vi "Avantes - take measurement.vi"(8 "error in (no error)":errorcluster, 10 "UI":refnum<queue>, 11 "Hardware Resources in":T1) -> (0 "error out":errorcluster, 2 "Spectral distribution out":cluster{dbl, dbl}[](graph), 3 "Hardware Resources out":T1)   [LabVIEW 2014, in "AvaSpec.lvlib" / "AvaSpec Acquisition.lvlib"]
doc: "Communicates the the spectrometer to perform measurements. The signal is sent to take a measurement with the corresponding measurement settings. The buffer is then polled for completed measurement data. Raw data is interpolated for integer frequencies, dark corrected, and analyzed for sensor saturation. If the full scale of the sensor isn't utilized optimally a more optimal integration time is itterated over. Once a measurement is taken that optimally uses the sensor range, the spectral distribution is outputted."
uses:
  AvaSpec Acquisition.lvlib
  Hardware Configuration.ctl
  Libraries/AS-5216-DLL/AVS settings.ctl
  Sphere Indicator.ctl
  Settings/Measurement Type.ctl
  support/Message Queue/Message Cluster.ctl
  support/Message Queue/Enqueue Message (Single).vi
  Libraries/AS-5216-DLL/Avantes Spectrometer Functions.lvlib
  support/Message Queue/AvaSpec Message Queue.lvlib
  Dark/Dark.lvlib
  AvaSpec.lvlib
panel:
  out "Raw Spectral distribution":cluster{dbl, dbl}[](graph)
  in  "force stop":bool
  out "i":i32
  # "Inputs"
  # "Out"
  # "Working"
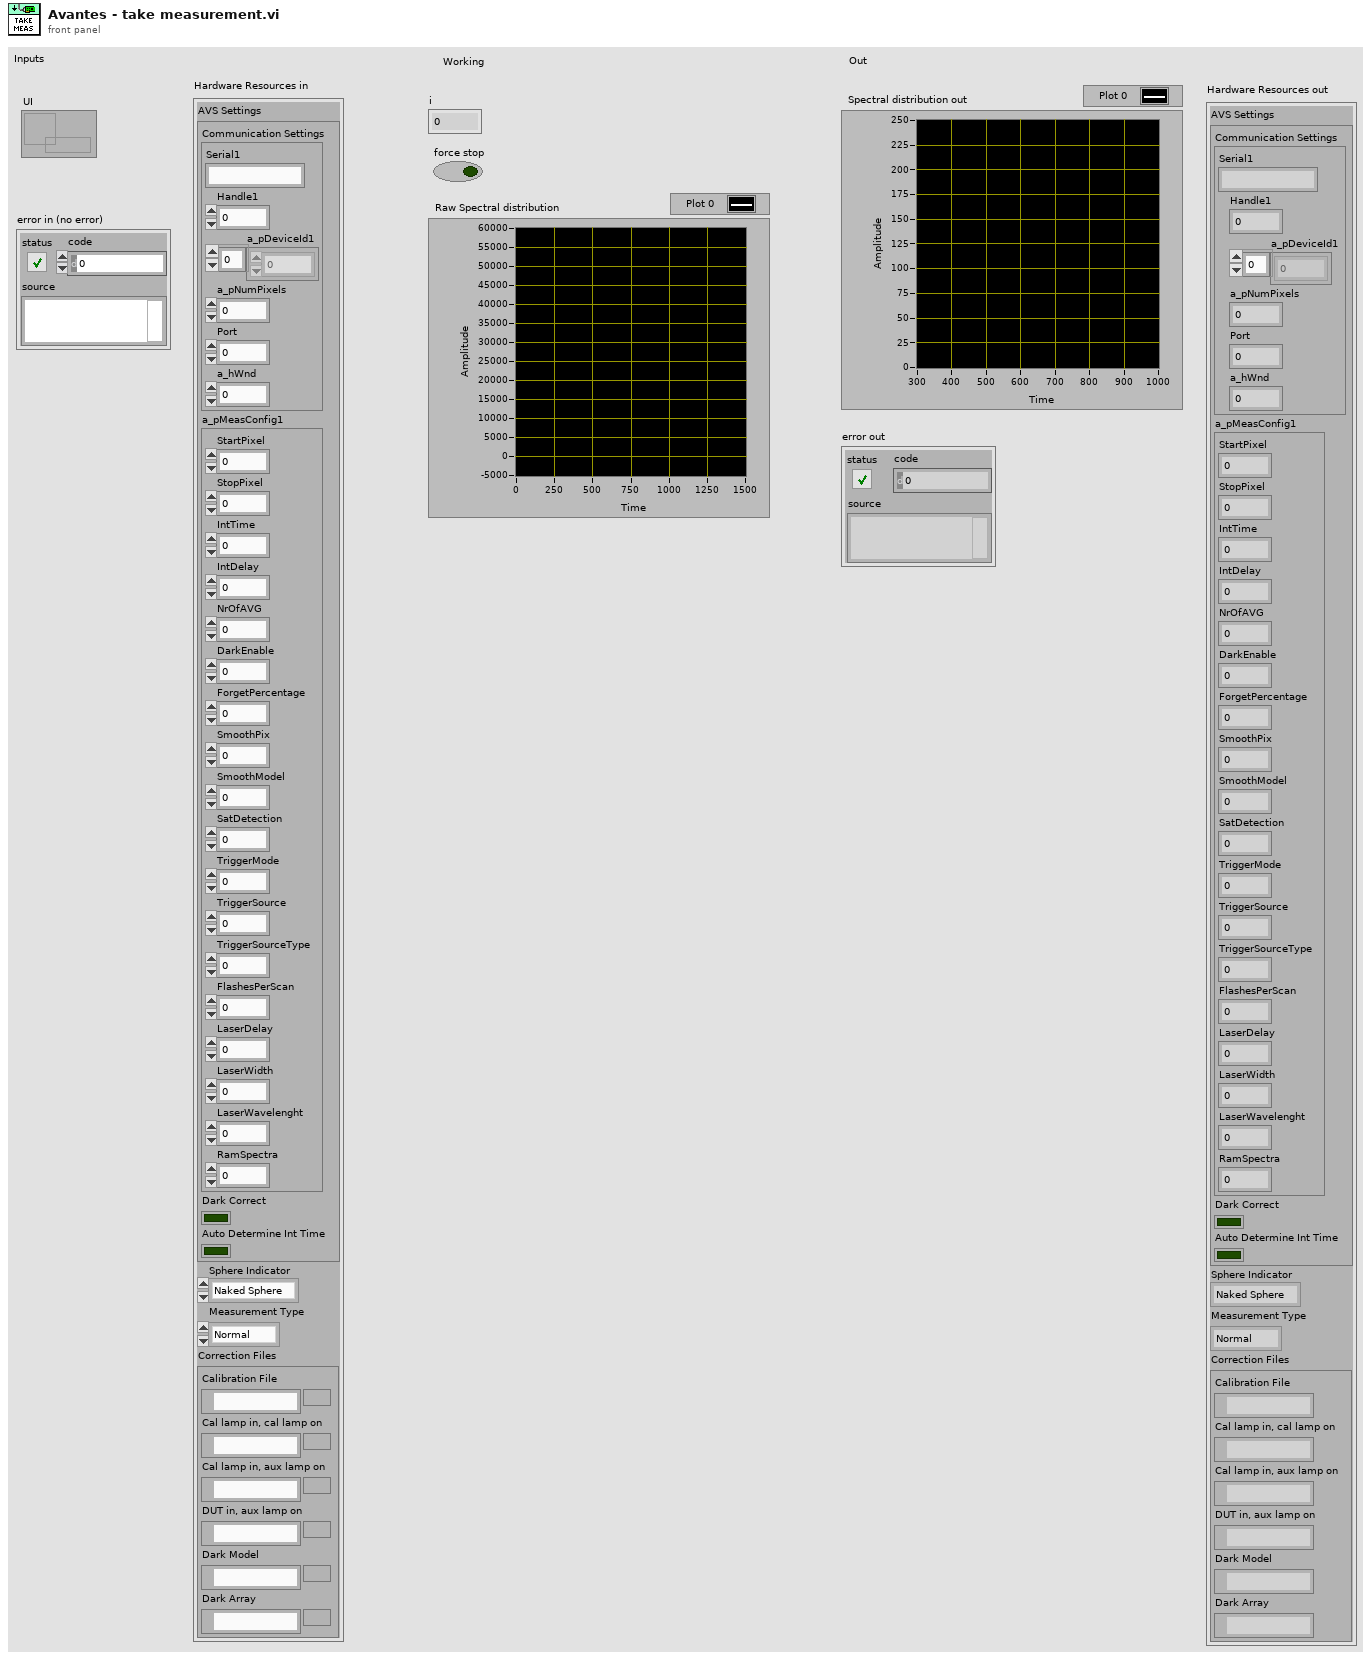
[diagram p1: front panel]
types:
  T1 = typedef "AvaSpec.lvlib/AvaSpec Acquisition.lvlib/Hardware Configuration.ctl" = cluster{"AVS Settings":T2, "Sphere Indicator":T3, "Measurement Type":T4, "Correction Files":cluster{"Calibration File":path, "Cal lamp in, cal lamp on":path, "Cal lamp in, aux lamp on":path, "DUT in, aux lamp on":path, "Dark Model":path, "Dark Array":path}}
  T2 = typedef "AvaSpec.lvlib/AVS settings.ctl" = cluster{"Communication Settings":cluster{"Serial1":string, "Handle1":i32, "a_pDeviceId1":u8[], "a_pNumPixels":u16, "Port":i32, "a_hWnd":i32}, "a_pMeasConfig1":cluster{"StartPixel":u16, "StopPixel":u16, "IntTime":sgl, "IntDelay":u32, "NrOfAVG":u32, "DarkEnable":u8, "ForgetPercentage":u8, "SmoothPix":u16, "SmoothModel":u8, "SatDetection":u8, "TriggerMode":u8, "TriggerSource":u8, "TriggerSourceType":u8, "FlashesPerScan":u16, "LaserDelay":u32, "LaserWidth":u32, "LaserWavelenght":sgl, "RamSpectra":u16}, "Dark Correct":bool, "Auto Determine Int Time":bool}
  T3 = typedef "AvaSpec.lvlib/Sphere Indicator.ctl" = enum16{"Naked Sphere", "Insulated Sphere"}
  T4 = typedef "AvaSpec.lvlib/AvaSpec Acquisition.lvlib/Measurement Type.ctl" = enum16{"Normal", "Calibration", "Dark"}
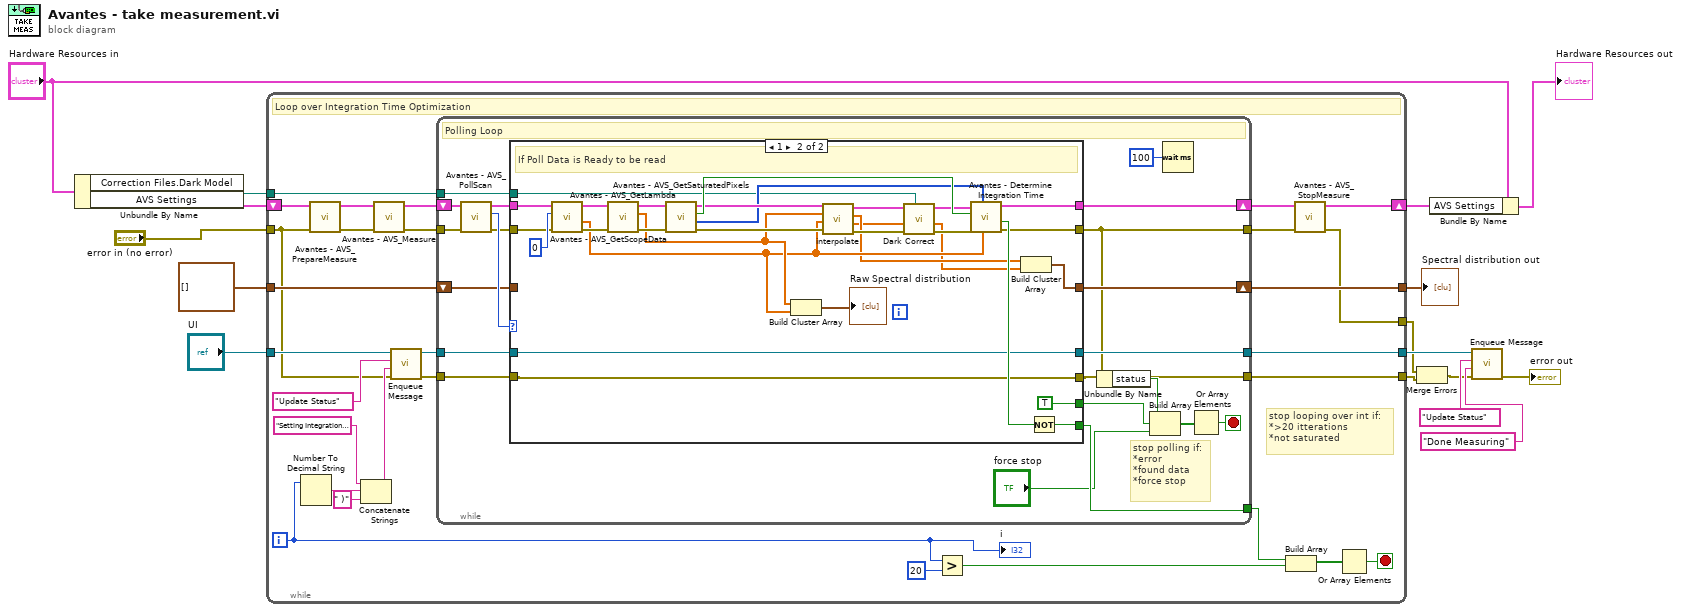
[diagram p0: block diagram]
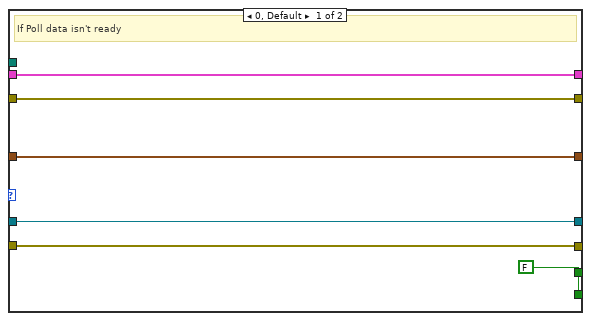
[diagram p2: hidden frame]
diagram:
  n1 = Unbundle By Name("Hardware Resources in") -> ("Correction Files.Dark Model"=w2:path, "AVS Settings"=w8:T2)
  n2 = while {
    tunnel: [w39] -> w4
    tunnel: [w45] -> w16
    tunnel: cluster{dbl, dbl}[] [] -> [w44]
    tunnel: "error in (no error)" -> [w19]
    shift-right: [w40] -> w6
    shift-left: w8 -> [w38]
    tunnel: "UI" -> [w33]
    tunnel: [w25] -> w12
    tunnel: w2 -> [w20]
    tunnel: [w17] -> w3
    i -> [w31]
    stop <- w21 stop-if-true
    # "stop looping over int if:\n*>20 itterations\n*not saturated"
    # "Loop over Integration Time Optimization"
    n3 = Number To Decimal String(number=w31) -> (decimal integer string=w29:string)  [unwired: 1 in]
    n4 = call "Avantes - AVS_PrepareMeasure.vi"("error in (no error)"=w19, "AVS Settings In"=w38) -> ("error out"=w36:errorcluster, "AVS Settings Out"=w37:T2)  [unwired: 8 in]
    n5 = Concatenate Strings("Setting Integration time ( " ("Message"), w29, " )" ("string")) -> (w27:string)
    n6 = call "Avantes - AVS_Measure.vi"("error in (no error)"=w36, "AVS Settings In"=w37) -> ("error out"=w35:errorcluster, "AVS Settings Out"=w34:T2)  [unwired: 8 in]
    n7 = call-poly "Enqueue Message.vi"("error in (no error)"=w19, "Message Data"=w27, "Message"="Update Status", "Message Queue"=w33) -> ("error out"=w18:errorcluster, "dup Message Queue"=w26:refnum<queue>)  [unwired: 6 in]
    n8 = while {
      tunnel: [w51] -> w41
      shift-right: [w63] -> w45
      shift-left: w44 -> [w61]
      shift-right: [w60] -> w43
      shift-left: w34 -> [w57]
      tunnel: [w59] -> w24
      tunnel: w35 -> [w58]
      tunnel: w26 -> [w56]
      tunnel: [w55] -> w25
      tunnel: w20 -> [w48]
      tunnel: w18 -> [w47]
      tunnel: [w46] -> w17
      stop <- w49 stop-if-true
      # "stop polling if:\n*error\n*found data\n*force stop"
      # "Polling Loop"
      n9 = call "Avantes - AVS_PollScan.vi"("error in (no error)"=w58, "AVS Settings In"=w57) -> ("error out"=w64:errorcluster, "Output Ready"=w66:i32, "AVS Settings Out"=w65:T2)  [unwired: 7 in]
      n10 = case shown="1" w66 {
        tunnel: w65 -> [w71 w81]
        tunnel: w64 -> [w72 w101]
        tunnel: [w72 w84] -> w51
        tunnel: [w70 w83] -> w63
        tunnel: [w69 TRUE] -> w52
        tunnel: [w71 w100] -> w60
        tunnel: w61 -> [w70 _]
        tunnel: [w69 w96] -> w59
        tunnel: w56 -> [w68 w95]
        tunnel: [w68 w95] -> w55
        tunnel: w48 -> [_ w87]
        tunnel: [w67 w82] -> w46
        tunnel: w47 -> [w67 w82]
        frame 0, Default {
          w69 = FALSE
          # "If Poll data isn't ready"
        }
        frame 1 {
          # "If Poll Data is Ready to be read"
          n11 = call "Avantes - AVS_GetScopeData.vi"("error in (no error)"=w101, "a_pTimeLabel"=u32 0, "AVS Settings In"=w81) -> ("error out"=w92:errorcluster, "a_pSpectrum"=w77:dbl[], "AVS Settings Out"=w80:T2)  [unwired: 5 in, 1 out]
          n12 = call "Avantes - AVS_GetLambda.vi"("error in (no error)"=w92, "AVS Settings In"=w80) -> ("error out"=w91:errorcluster, "a_pWaveLength"=w78:dbl[], "AVS Settings Out"=w79:T2)  [unwired: 7 in]
          n13 = call "Avantes - AVS_GetSaturatedPixels.vi"("error in (no error)"=w91, "AVS Settings In"=w79) -> ("error out"=w94:errorcluster, "a_pSaturated"=w89:u8[], "Saturated?"=w99:bool, "AVS Settings Out"=w90:T2)  [unwired: 6 in]
          n14 = Build Cluster Array(w78, w77) -> (→"Raw Spectral distribution":cluster{dbl, dbl}[])
          n15 = call "interpolate.vi"("error in (no error)"=w94, "a_pSpectrum"=w77, "a_pWaveLength"=w78, "AVS Settings In"=w90) -> ("error out"=w93:errorcluster, "Counts Out"=w74:dbl[], "Wavelengths Out"=w76:dbl[], "AVS Settings out"=w88:T2)  [unwired: 4 in]
          n16 = call "Dark Correct.vi"("Dark Array Model Path"=w87, "error in (no error)"=w93, "Counts"=w74, "AVS Settings In"=w88) -> ("error out"=w86:errorcluster, "Counts normalize and dark corrected"=w73:dbl[], "AVS Settings Out"=w85:T2)  [unwired: 5 in]
          n17 = call "Avantes - Determine Integration Time.vi"("a_pSpectrum"=w77, "a_pSaturated"=w89, "error in (no error)"=w86, "Saturated?"=w99, "AVS Settings In"=w85) -> ("error out"=w84:errorcluster, "Continue Int Time Seek"=w98:bool, "AVS Settings Out"=w100:T2)  [unwired: 4 in]
          n18 = Build Cluster Array(w76, w73) -> (w83:cluster{"Numeric":dbl, dbl}[])
          n19 = Not(x=w98) -> (.not. x?=w96:bool)
        }
      }
      n20 = Unbundle By Name(w51) -> ("status"=w50:bool)
      n21 = Build Array(w50, w52, "force stop") -> (w54:bool[])
      n22 = Wait (ms)(milliseconds to wait=u32 100) -> ()  [unwired: 1 out]
      n23 = Or Array Elements(Boolean array=w54) -> (logical OR=w49:bool)
    }
    n24 = Greater?(x=w31, y=20) -> (0:w23:bool)
    n25 = Build Array(w24, w23) -> (w22:bool[])
    n26 = call "Avantes - AVS_StopMeasure.vi"("error in (no error)"=w41, "AVS Settings In"=w43) -> ("error out"=w39:errorcluster, "AVS Settings Out"=w40:T2)  [unwired: 8 in]
    n27 = Or Array Elements(Boolean array=w22) -> (logical OR=w21:bool)
    "i" <- w31
  }
  "Spectral distribution out" <- w16
  n28 = Merge Errors(w4, w3) -> (w5:errorcluster)
  n29 = Bundle By Name(cluster="Hardware Resources in", "AVS Settings"=w6) -> (→"Hardware Resources out":T1)
  n30 = call-poly "Enqueue Message.vi"("error in (no error)"=w5, "Message Data"="Done Measuring" ("Message"), "Message"="Update Status", "Message Queue"=w12) -> ("error out"=→"error out":errorcluster)  [unwired: 6 in, 1 out]
